vi "Measurement Logic.vi"(8 "error in":errorcluster, 10 "Measurement Context":refnum<class "MeasurementContext.lvclass">, 11 "Measurement Configuration":T2={"Victim channel"=0, "Full scale range"=10.0, "Interferer channels"=[2], "Victim channel resource name"="", "Victim frequency"=-1.0, "Victim amplitude"=1000.0, "Interferer channel resource name"="", "Interferer channel channel"=0, "Interferer start frequency"=100000.0, "Interferer stop frequency"=160000.0, "Interferer number of steps"=10, "Interferer sweep type"=0, "Interferer amplitude"=-1.0, "Digital capture resource name"="", "Digital capture sample rate"=800000.0, "Digital capture samples"=800000} {"Interferer sweep type" items=["Linear", "Logarithmic"]}) -> (0 "error out":errorcluster, 2 "Measurement Context out":refnum<class "MeasurementContext.lvclass">, 3 "Measurement Results":T1)   [LabVIEW 2021, in "adc_chToChIsolationMeasurement.lvlib"]
uses:
  adc_chToChIsolationMeasurement.lvlib
  Measurement Configuration.ctl
  Measurement Results.ctl
  <vilib>/MeasurementLink/MeasurementLink Measurement Server/Classes/MeasurementContext/MeasurementContext.lvclass
  <vilib>/gRPC/LabVIEW gRPC Library/Shared/grpcId.ctl
  shared/controls/HW Sync Commands.ctl
  <instrlib>/niFgen/niFgen.llb/niFgen Waveform Type.ctl
  <instrlib>/niFgen/niFgen.llb/niFgen Output Mode.ctl
  <vilib>/DAQmx/create/channels.llb/DAQmx Create Channel (AO-Voltage-Basic).vi
  <vilib>/DAQmx/configure/timing.llb/DAQmx Timing (Sample Clock).vi
  shared/digitalInterface/client/dcvmDPI_AD7606B_client/dcvmDPI_AD7606B_client.lvlib
  shared/digitalInterface/client/dcvmDPI_AD7606B_clientImpl/dcvmDPI_AD7606B_clientImpl.lvlib
  <vilib>/gRPC/LabVIEW gRPC Library/grpc-lvsupport-release.lvlib
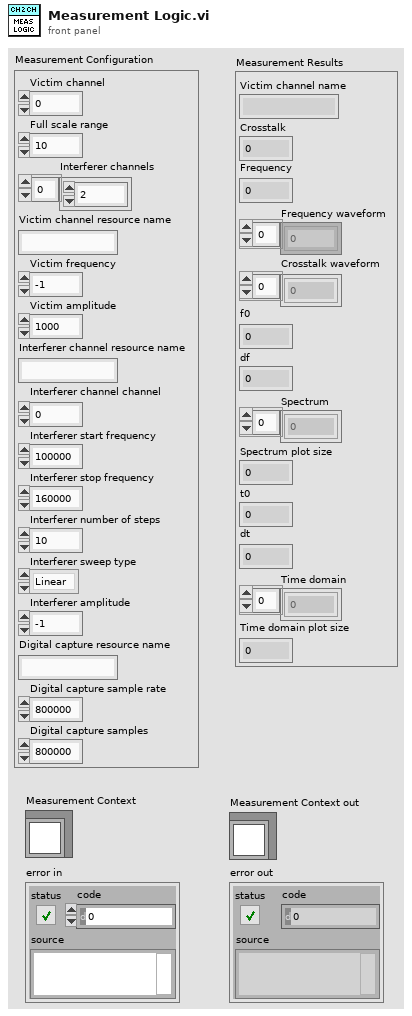
[diagram p1: front panel]
types:
  T1 = typedef "adc_chToChIsolationMeasurement.lvlib/Measurement Results.ctl" = cluster{"Victim channel name":string, "Crosstalk":dbl, "Frequency":dbl, "Frequency waveform":dbl[], "Crosstalk waveform":dbl[], "f0":dbl, "df":dbl, "Spectrum":dbl[], "Spectrum plot size":i32, "t0":dbl, "dt":dbl, "Time domain":dbl[], "Time domain plot size":i32}
  T2 = typedef "adc_chToChIsolationMeasurement.lvlib/Measurement Configuration.ctl" = cluster{"Victim channel":i32, "Full scale range":dbl, "Interferer channels":i32[], "Victim channel resource name":string, "Victim frequency":dbl, "Victim amplitude":dbl, "Interferer channel resource name":string, "Interferer channel channel":i32, "Interferer start frequency":dbl, "Interferer stop frequency":dbl, "Interferer number of steps":i32, "Interferer sweep type":u16, "Interferer amplitude":dbl, "Digital capture resource name":string, "Digital capture sample rate":dbl, "Digital capture samples":u32}
  T3 = typedef "HW Sync Commands.ctl" = enum16{"NoAction", "GenerationStarted", "AcquisitionCompleted", "GenerationErrored"}
  T4 = typedef "grpc-lvsupport-release.lvlib/grpcId.ctl" = u64
  T5 = cluster{"DSG Session":refnum<k21>, "FGen Session":refnum<k15>, "gRPC session":T4}
  T6 = typedef "niFgen Output Mode.ctl" = u32
  T7 = typedef "niFgen Waveform Type.ctl" = i32
  T8 = typedef "Sync Commands.ctl" = enum16{"NoAction", "GenerationStarted", "AcquisitionCompleted", "GenerationErrored"}
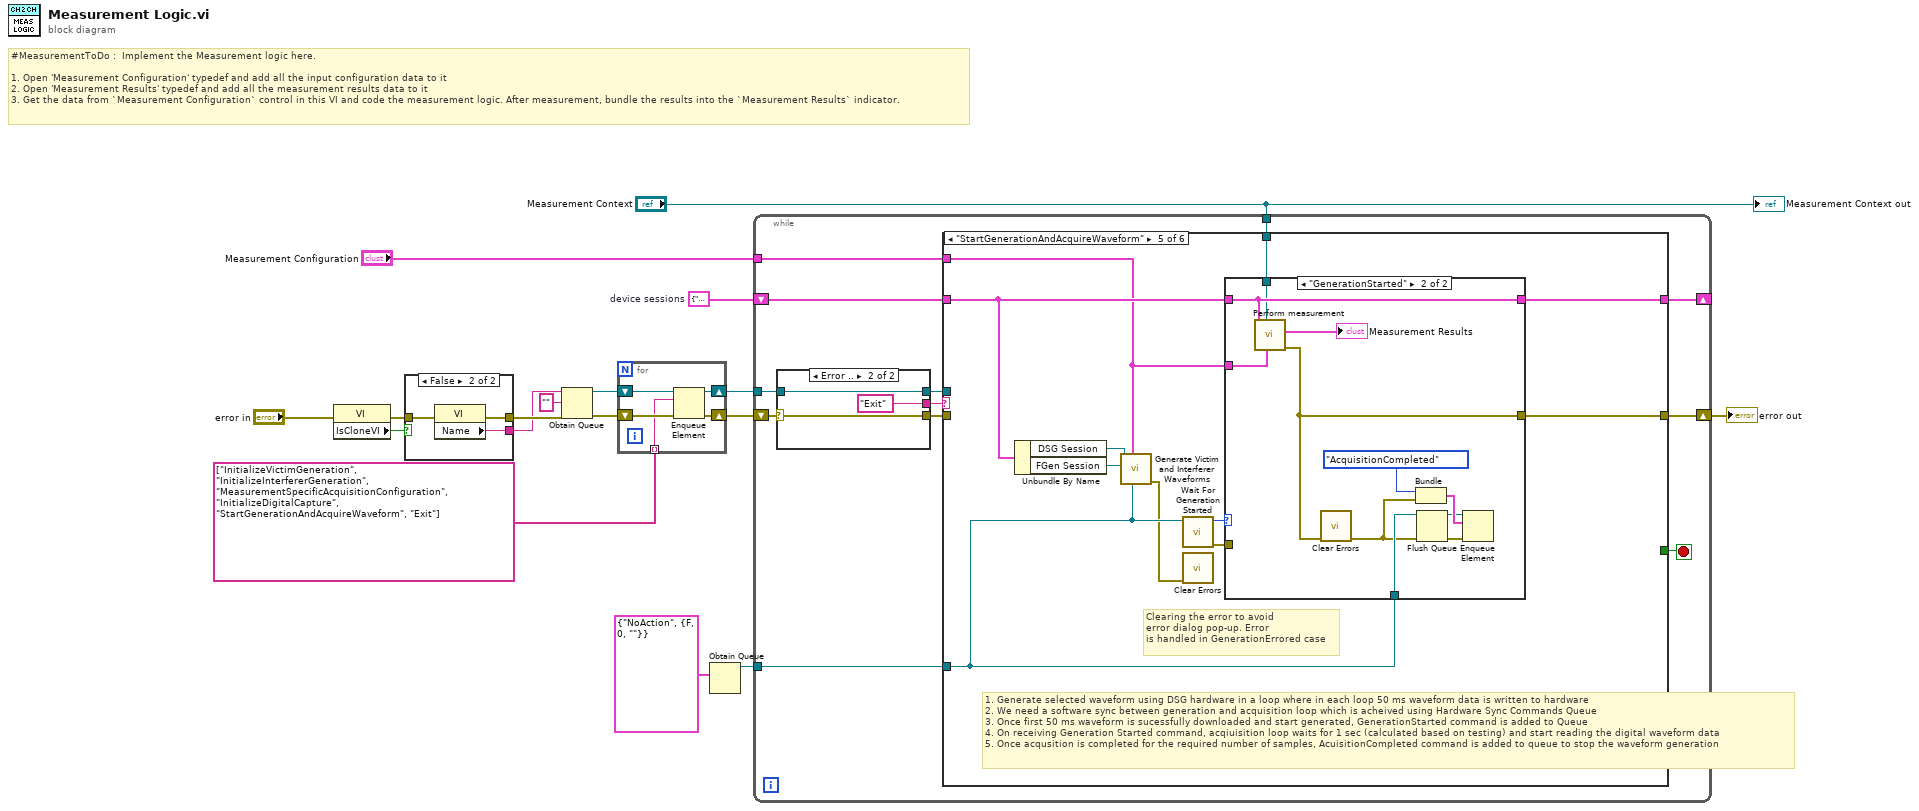
[diagram p0: block diagram]
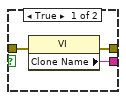
[diagram p2: hidden frame]
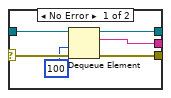
[diagram p3: hidden frame]
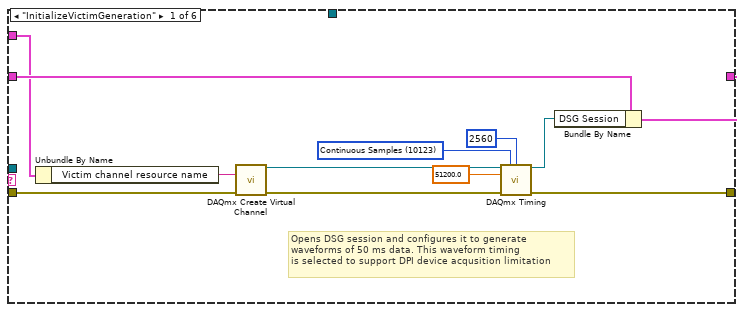
[diagram p4: hidden frame]
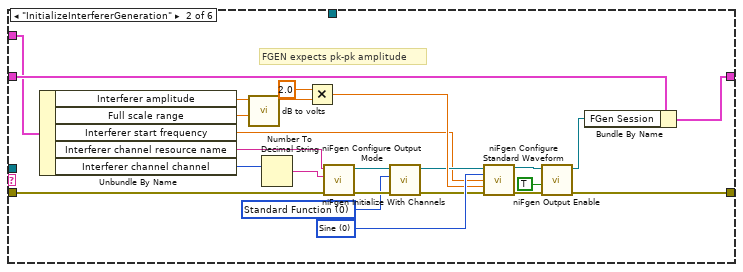
[diagram p5: hidden frame]
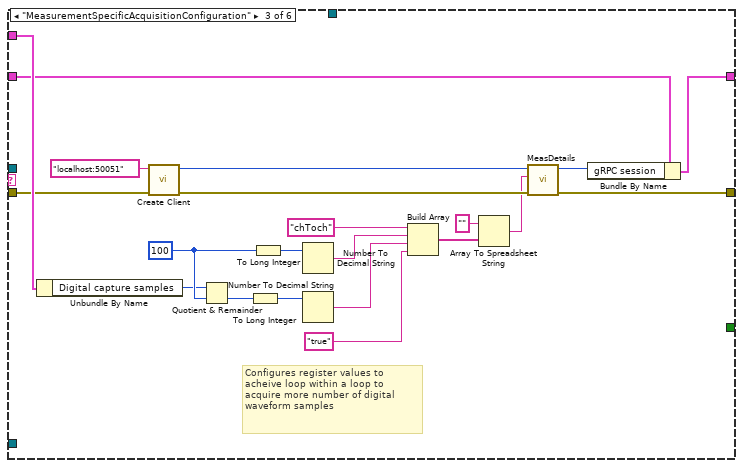
[diagram p6: hidden frame]
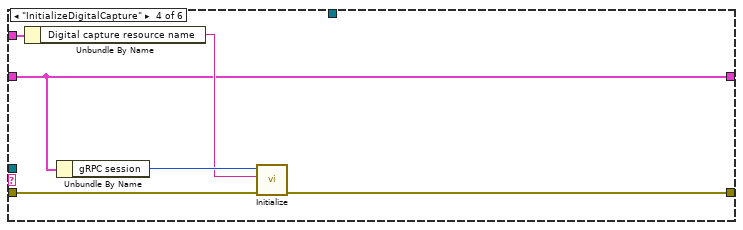
[diagram p7: hidden frame]
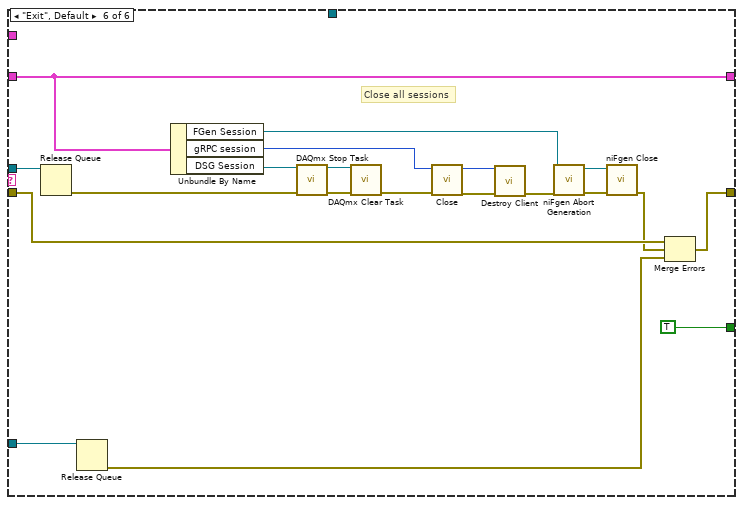
[diagram p9: hidden frame]
diagram:
  w14 = T5 {"DSG Session"="", "FGen Session"="", "gRPC session"=0}  # device sessions
  # "#MeasurementToDo :  Implement the Measurement logic here.\n\n1. Open 'Measurement Configuration' typedef and add all the input configuration data to it\n2. Open 'Measurement Results' typedef and add all the measurement results data to it\n3. Get the data from `Measurement Configuration` control in this VI and code the measurement logic. After measurement, bundle the results into the `Measurement Results` indicator."
  n1 = property class="VI"(error in="error in") -> (error out=w8:errorcluster, "IsCloneVI"=w9:bool)  [unwired: 1 in, 1 out]
  n2 = case shown="False" w9 {
    tunnel: [w20 w23] -> w6
    tunnel: [w19 w22] -> w5
    tunnel: w8 -> [w18 w21]
    frame True {
      n3 = property class="VI"(error in=w18) -> (error out=w20:errorcluster, "Clone Name"=w19:string)  [unwired: 1 in, 1 out]
    }
    frame False {
      n4 = property class="VI"(error in=w21) -> (error out=w23:errorcluster, "Name"=w22:string)  [unwired: 1 in, 1 out]
    }
  }
  n5 = Obtain Queue(name (unnamed)=w5, element data type="", error in (no error)=w6) -> (queue out=w16:refnum<queue>, error out=w4:errorcluster)  [unwired: 2 in, 1 out]
  n6 = for {
    shift-right: [w26] -> w15
    shift-left: w16 -> [w28]
    shift-right: [w25] -> w3
    shift-left: w4 -> [w27]
    tunnel: string[] ["InitializeVictimGeneration", "InitializeInterfererGeneration", "MeasurementSpecificAcquisitionConfiguration", "InitializeDigitalCapture", "StartGenerationAndAcquireWaveform", "Exit"] ("Step sequence") -> [w24] mode=indexing
    n7 = Enqueue Element(queue=w28, element=w24, error in (no error)=w27) -> (queue out=w26:refnum<queue>, error out=w25:errorcluster)  [unwired: 1 in, 1 out]
  }
  n8 = Obtain Queue(element data type=cluster{"Status":T3, "Error":errorcluster} {"Status"=enum."NoAction", "Error"={"status"=FALSE, "code"=0, "source"=""}}) -> (queue out=w12:refnum<queue>)  [unwired: 4 in, 2 out]
  n9 = while {
    tunnel: w15 -> [w33]
    shift-right: [w40] -> w10
    shift-left: w3 -> [w34]
    tunnel: "Measurement Configuration" -> [w38]
    shift-right: [w36] -> _
    shift-left: w14 -> [w37]
    tunnel: w12 -> [w35]
    tunnel: "Measurement Context" -> [w29]
    stop <- w39 stop-if-true
    n10 = case shown="Error .." w34 {
      selector: w34 -> [w44 w48]
      tunnel: w33 -> [w46 w47]
      tunnel: [w45 "Exit" ("t")] -> w32
      tunnel: [w43 w48] -> w31
      tunnel: [w41 w47] -> w30
      frame No Error {
        n11 = Dequeue Element(queue=w46, timeout in ms (-1)=100, error in (no error)=w44) -> (queue out=w41:refnum<queue>, element=w45:string, error out=w43:errorcluster)  [unwired: 1 out]
      }
      frame Error {
      }
    }
    n12 = case shown="\"StartGenerationAndAcquireWaveform\"" w32 {
      tunnel: [w59 w69 w90 w107 w123 w147] -> w40
      tunnel: w31 -> [w60 w81 w94 w110 _ w148]
      tunnel: [_ _ _ _ _ TRUE] -> w39
      tunnel: w38 -> [w56 w83 w105 w112 w116 _]
      tunnel: w37 -> [w58 w85 w88 w108 w122 w152]
      tunnel: [w57 w84 w86 w108 w121 w152] -> w36
      tunnel: w35 -> [_ _ _ _ w120 w151]
      tunnel: w30 -> [_ _ _ _ _ w150]
      tunnel: w29 -> [_ _ _ _ w113 _]
      frame "InitializeVictimGeneration" {
        w52 = 10123 items=["Finite Samples"=10178, "Continuous Samples"=10123, "Hardware Timed Single Point"=12522] ("sample mode")
        # "Opens DSG session and configures it to generate\nwaveforms of 50 ms data. This waveform timing\nis selected to support DPI device acqusition limitation"
        n13 = Unbundle By Name(w56) -> ("Victim channel resource name"=w61:string)
        n14 = call-poly <vilib>:"DAQmx Create Virtual Channel.vi"("physical channels"=w61, "error in"=w60) -> ("task out"=w54:refnum<k21>, "error out"=w53:errorcluster)  [unwired: 12 in]
        n15 = call-poly <vilib>:"DAQmx Timing.vi"("task/channels in"=w54, "sample mode"=w52, "samples per channel"=2560, "rate"=51200.0, "error in"=w53) -> ("task out"=w55:refnum<k21>, "error out"=w59:errorcluster)  [unwired: 9 in]
        n16 = Bundle By Name(cluster=w58, "DSG Session"=w55) -> (w57:T5)
      }
      frame "InitializeInterfererGeneration" {
        w73 = T6 0 items=["Standard Function", "Frequency List", "Arbitrary Waveform", "Arbitrary Sequence", "Script"] ("Output Mode (default: 0=Standard Function)")
        w80 = T7 0 items=["Sine", "Square", "Triangle", "Ramp Up", "Ramp Down", "DC", "Noise", "User"] ("Waveform")
        # "FGEN expects pk-pk amplitude"
        n17 = Unbundle By Name(w83) -> ("Interferer amplitude"=w67:dbl, "Full scale range"=w64:dbl, "Interferer start frequency"=w65:dbl, "Interferer channel resource name"=w82:string, "Interferer channel channel"=w63:i32)
        n18 = call "dB to volts.vi"("Full scale range"=w64, "Voltage(dB)"=w67) -> ("Voltage(volts)"=w66:dbl)  [unwired: 9 in]
        n19 = Number To Decimal String(number=w63) -> (decimal integer string=w62:string)  [unwired: 1 in]
        n20 = Multiply(x=2.0 ("y"), y=w66) -> (x*y=w79:dbl)
        n21 = call <instrlib>:"niFgen Initialize With Channels.vi"("error in (no error)"=w81, "Channel Name"=w62, "Resource Name"=w82) -> ("error out"=w75:errorcluster, "Instrument Handle Out"=w77:refnum<k15>)  [unwired: 7 in]
        n22 = call <instrlib>:"niFgen Configure Output Mode.vi"("error in (no error)"=w75, "Output Mode (default: 0=Standard Function)"=w73, "Instrument Handle"=w77) -> ("error out"=w74:errorcluster, "Instrument Handle Out"=w76:refnum<k15>)  [unwired: 6 in]
        n23 = call <instrlib>:"niFgen Configure Standard Waveform.vi"("Instrument Handle"=w76, "Waveform"=w80, "Frequency"=w65, "Amplitude"=w79, "error in (no error)"=w74) -> ("Instrument Handle Out"=w72:refnum<k15>, "error out"=w70:errorcluster)  [unwired: 9 in]
        n24 = call <instrlib>:"niFgen Output Enable.vi"("error in (no error)"=w70, "Output Enable (default: True)"=TRUE, "Instrument Handle"=w72) -> ("error out"=w69:errorcluster, "Instrument Handle Out"=w71:refnum<k15>)  [unwired: 7 in]
        n25 = Bundle By Name(cluster=w85, "FGen Session"=w71) -> (w84:T5)
      }
      frame "MeasurementSpecificAcquisitionConfiguration" {
        w106 = u32 100 ("value")
        # "Configures register values to acheive loop within a loop to acquire more number of digital waveform samples"
        n26 = Unbundle By Name(w105) -> ("Digital capture samples"=w104:u32)
        n27 = call "Create Client.vi"("error in"=w94, "address"="localhost:50051") -> ("error out"=w91:errorcluster, "gRPC ID Out"=w92:T4)  [unwired: 8 in]
        n28 = Quotient & Remainder(x=w104, y=w106) -> (floor(x/y)=w103:u32)  [unwired: 1 out]
        n29 = To Long Integer(number=w103) -> (32bit integer=w101:i32)
        n30 = To Long Integer(number=w106) -> (32bit integer=w102:i32)
        n31 = Number To Decimal String(number=w102) -> (decimal integer string=w99:string)  [unwired: 1 in]
        n32 = Number To Decimal String(number=w101) -> (decimal integer string=w98:string)  [unwired: 1 in]
        n33 = Build Array("chToch", w99, w98, "true") -> (w96:string[])
        n34 = Array To Spreadsheet String(array=w96, 3:"" ("format string")) -> (spreadsheet string=w89:string)  [unwired: 1 in]
        n35 = call "MeasDetails.vi"("error in"=w91, "Active measurement"=w89, "gRPC session in"=w92) -> ("error out"=w90:errorcluster, "gRPC session out"=w87:T4)  [unwired: 7 in]
        n36 = Bundle By Name(cluster=w88, "gRPC session"=w87) -> (w86:T5)
      }
      frame "InitializeDigitalCapture" {
        n37 = Unbundle By Name(w112) -> ("Digital capture resource name"=w109:string)
        n38 = Unbundle By Name(w108) -> ("gRPC session"=w111:T4)
        n39 = call "Initialize.vi"("error in"=w110, "Digital capture resource name"=w109, "gRPC session in"=w111) -> ("error out"=w107:errorcluster)  [unwired: 7 in, 1 out]
      }
      frame "StartGenerationAndAcquireWaveform" {
        # "1. Generate selected waveform using DSG hardware in a loop where in each loop 50 ms waveform data is written to hardware\n2. We need a software sync between generation and acquisition loop which is acheived using Hardware Sync Commands Queue\n3. Once first 50 ms waveform is sucessfully downloaded and start generated, GenerationStarted command is added to Queue\n4. On receiving Generation Started command, acqiuisition loop waits for 1 sec (calculated based on testing) and start reading the digital waveform data\n5. Once acqusition is completed for the required number of samples, AcuisitionCompleted command is added to queue to stop the waveform generation"
        # "Clearing the error to avoid\nerror dialog pop-up. Error\nis handled in GenerationErrored case"
        n40 = Unbundle By Name(w122) -> ("DSG Session"=w115:refnum<k21>, "FGen Session"=w114:refnum<k15>)
        n41 = call "Generate Victim and Interferer Waveforms.vi"("hardware commands sync queue"=w120, "measurement configuration"=w116, "FGen session in"=w114, "DSG task in"=w115) -> ("error out"=w117:errorcluster)  [unwired: 7 in]
        n42 = call "Wait For Generation Started.vi"("hardware commands sync queue"=w120) -> ("error out"=w118:errorcluster, "Status"=w119:T8)  [unwired: 9 in]
        n43 = call <vilib>:"Clear Errors.vi"("error in (no error)"=w117) -> ()  [unwired: 5 in, 2 out]
        n44 = case shown="\"GenerationStarted\"" w119 {
          tunnel: [w124 w128] -> w123
          tunnel: w120 -> [_ w133]
          tunnel: w122 -> [w125 w127]
          tunnel: [w125 w127] -> w121
          tunnel: w116 -> [_ w130]
          tunnel: w118 -> [w124 _]
          tunnel: w113 -> [_ w126]
          frame Default {
          }
          frame "GenerationStarted" {
            n45 = call "Perform measurement.vi"("measurement configuration"=w130, "Measurement Context"=w126, "device sessions"=w127) -> ("error out"=w128:errorcluster, "measurement results"=→"Measurement Results":T1)  [unwired: 7 in]
            n46 = call <vilib>:"Clear Errors.vi"("error in (no error)"=w128) -> ("error out"=w132:errorcluster)  [unwired: 5 in, 1 out]
            n47 = Bundle("element"=HW_Sync_Commands."AcquisitionCompleted", "error out"=w132) -> (w135:cluster{"element":T3, "error out":errorcluster})  [unwired: 1 in]
            n48 = Flush Queue(queue=w133, error in (no error)=w132) -> (queue out=w134:refnum<queue>, error out=w131:errorcluster)  [unwired: 1 out]
            n49 = Enqueue Element(queue=w134, element=w135, error in (no error)=w131) -> ()  [unwired: 1 in, 3 out]
          }
        }
      }
      frame "Exit", Default {
        # "Close all sessions"
        n50 = Release Queue(queue=w150) -> (error out=w149:errorcluster)  [unwired: 2 in, 2 out]
        n51 = Release Queue(queue=w151) -> (error out=w146:errorcluster)  [unwired: 2 in, 2 out]
        n52 = Unbundle By Name(w152) -> ("FGen Session"=w143:refnum<k15>, "gRPC session"=w141:T4, "DSG Session"=w155:refnum<k21>)
        n53 = call <vilib>:"DAQmx Stop Task.vi"("task/channels in"=w155, "error in"=w149) -> ("task out"=w154:refnum<k21>, "error out"=w153:errorcluster)  [unwired: 12 in]
        n54 = call <vilib>:"DAQmx Clear Task.vi"("task in"=w154, "error in"=w153) -> ("error out"=w140:errorcluster)  [unwired: 13 in]
        n55 = call "Close.vi"("error in"=w140, "gRPC session in"=w141) -> ("error out"=w138:errorcluster, "gRPC session out"=w139:T4)  [unwired: 8 in]
        n56 = call "Destroy Client.vi"("error in"=w138, "gRPC ID"=w139) -> ("error out"=w137:errorcluster)  [unwired: 9 in]
        n57 = call <instrlib>:"niFgen Abort Generation.vi"("error in (no error)"=w137, "Instrument Handle"=w143) -> ("error out"=w144:errorcluster, "Instrument Handle Out"=w142:refnum<k15>)  [unwired: 8 in]
        n58 = call <instrlib>:"niFgen Close.vi"("error in (no error)"=w144, "Instrument Handle"=w142) -> ("error out"=w145:errorcluster)  [unwired: 9 in]
        n59 = Merge Errors(w148, w145, w146) -> (w147:errorcluster)
      }
    }
  }
  "error out" <- w10
  "Measurement Context out" <- "Measurement Context"
